vi "Lookup Child by Name.vi"(8 "error in (no error)":errorcluster, 10 "Name":string, 11 "Config Element in":refnum<class "Config Element.lvclass">) -> (0 "error out":errorcluster, 1 "Found":bool, 2 "Child":refnum<class "Config Element.lvclass">, 3 "Config Element out":refnum<class "Config Element.lvclass">)   [LabVIEW 2020, in "CDM-Config.lvlib" / "Config Element.lvclass"]
doc: "Looks up a direct child by name. If it is not found an error is returned."
uses:
  Config Element.lvclass
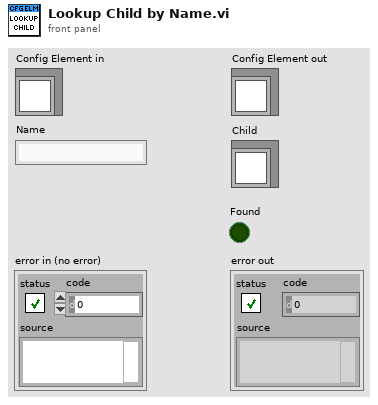
[diagram p1: front panel]
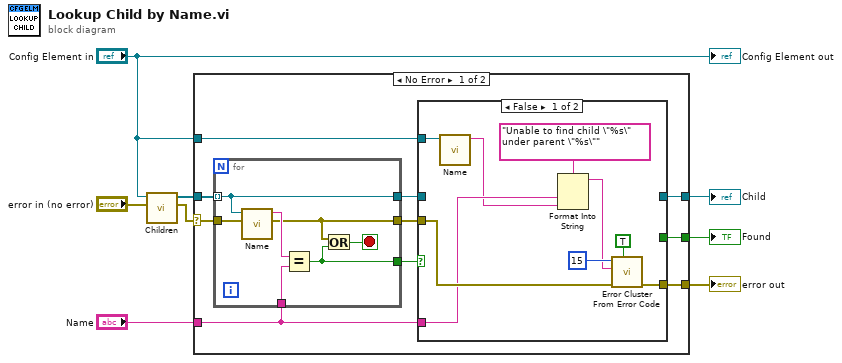
[diagram p0: block diagram]
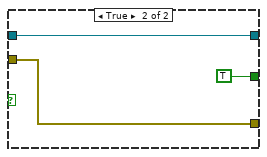
[diagram p2: hidden frame]
diagram:
  n1 = call "Children.vi"("error in (no error)"="error in (no error)", "Config Element in"="Config Element in") -> ("error out"=w7:errorcluster, "Elements"=w6:refnum<class "Config Element.lvclass">[])  [unwired: 8 in]
  n2 = case shown="No Error" w7 {
    selector: w7 -> [w17 w38]
    tunnel: w6 -> [w18 _]
    tunnel: "Name" -> [w12 _]
    tunnel: [w15 _] -> w4
    tunnel: "Config Element in" -> [w11 _]
    tunnel: [w10 w38] -> w2
    tunnel: [w9 _] -> w1
    frame No Error {
      n3 = for {
        tunnel: w18 -> [w34] mode=indexing
        tunnel: w17 -> [w37]
        tunnel: w12 -> [w36]
        tunnel: [w34] -> w14
        tunnel: [w33] -> w16
        tunnel: [w31] -> w13
        stop <- w32 stop-if-true
        n4 = call "Name.vi"("error in (no error)"=w37, "Config Element in"=w34) -> ("error out"=w31:errorcluster, "Name"=w35:string)  [unwired: 8 in]
        n5 = Equal?(x=w35, y=w36) -> (x = y?=w33:bool)
        n6 = Or(x=w31, y=w33) -> (x .or. y?=w32:bool)
      }
      n7 = case shown="False" w16 {
        tunnel: [_ w30] -> w15
        tunnel: w14 -> [_ w30]
        tunnel: w13 -> [w26 w28]
        tunnel: w12 -> [w22 _]
        tunnel: w11 -> [w25 _]
        tunnel: [w19 w28] -> w10
        tunnel: [_ TRUE] -> w9
        frame False {
          n8 = call "Name.vi"("Config Element in"=w25) -> ("Name"=w21:string)  [unwired: 9 in, 1 out]
          n9 = Format Into String(format string="Unable to find child \"%s\" under parent \"%s\"", w22, w21) -> (resulting string=w20:string)  [unwired: 2 in, 1 out]
          n10 = call <vilib>:"Error Cluster From Error Code.vi"("show call chain? (False)"=TRUE, "error in (no error)"=w26, "error message (\"\")"=w20, "error code (0)"=15) -> ("error out"=w19:errorcluster)  [unwired: 5 in]
        }
        frame True {
        }
      }
    }
    frame Error {
    }
  }
  "error out" <- w2
  "Child" <- w4
  "Found" <- w1
  "Config Element out" <- "Config Element in"
